vi "SERIAL_BufferLoopEx.vi"(11 "navX DevRef":T1={"SerialPortRef"={"DevStatus"={"status"=FALSE, "code"=0, "source"=""}, "Serial Port Name"=""}, "Board Information"={"WhoAmI (50 | 0x32)"=0, "Board Revision"=0, "Firmware Major Version"=0, "Firmware Minor Version"=0, "NAVX_BOARD_CAPABILITY"={"OMNIMOUNT"=FALSE, "YAW_RESET"=FALSE, "VEL_AND_DISP"=FALSE}, "NAVX_BOARD_YAW_AXIS"={"BOARD_YAW_AXIS_UP"=FALSE, "BOARD_YAW_AXIS"=0}}, "Status"={"Update Rate Hz"=0, "Accelerometer Full-Scale Range"=0, "Gyro Full-Scale Range"=0, "NAVX_OP_STATUS"=0, "NAVX_CAL_STATUS"=0, "NAVX_SELFTEST_STATUS"=0, "NAVX_SENSOR_STATUS"={"MOVING"=FALSE, "YAW_STABLE"=FALSE, "MAG_DISTURBANCE"=FALSE, "ALTITUDE_VALID"=FALSE, "SEALEVEL_PRESS_SET"=FALSE, "FUSED_HEADING_VALID"=FALSE}}, "Offsets"={"Yaw"=0.0, "Quat W"=0.0, "Quat X"=0.0, "Quat Y"=0.0, "Quat Z"=0.0}, "Update Rate (4Hz-60Hz)"=50, "Nav6Mode (YPR)"=enum."YPR", "refnum name"="", "error"={"status"=FALSE, "code"=0, "source"=""}, "Loop VI Refnum"=refnum, "Serial Port"=enum."Onboard RS-232"} {"Status"."NAVX_OP_STATUS" items=["INITIALIZING", "SELFTEST_IN_PROGRESS", "ERROR", "IMU_AUTOCAL_IN_PROGRESS", "NORMAL"]; "Status"."NAVX_CAL_STATUS" items=["IMU_CAL_STATE_MASK"=3, "IMU_CAL_INPROGRESS"=0, "IMU_CAL_ACCUMULATE"=1, "IMU_CAL_COMPLETE"=2, "MAG_CAL_COMPLETE"=4, "BARO_CAL_COMPLETE"=8]}) -> ()   [LabVIEW 2014, in "navX-MXP IMU.lvlib"]
uses:
  navX-MXP IMU.lvlib
  Internal/navX Serial DevRef.ctl
  <vilib>/Rock Robotics/WPI/SerialPort/WPI_SerialPortRef.ctl
  COMMON/TypeDefs/Data TypeDefs/navX Board Information.ctl
  COMMON/TypeDefs/Value TypeDefs/navX NAVX_BOARD_CAPABILITY.ctl
  COMMON/TypeDefs/Value TypeDefs/navX NAVX_BOARD_YAW_AXIS.ctl
  COMMON/TypeDefs/Data TypeDefs/navX Status Data.ctl
  COMMON/TypeDefs/Value TypeDefs/navX NAVX_OP_STATUS.ctl
  COMMON/TypeDefs/Value TypeDefs/navX NAVX_CAL_STATUS.ctl
  COMMON/TypeDefs/Value TypeDefs/navX NAVX_SENSOR_STATUS.ctl
  TypeDefs/navX Serial Mode.ctl
  NI WPI/WPI_SerialPort_USB.ctl
  TypeDefs/navX Data Packet ID.ctl
  <vilib>/Platform/TimedLoop/XDataNode/timing_clust.ctl
  <vilib>/Platform/TimedLoop/XDataNode/nitl_modes.ctl
  <vilib>/Platform/TimedLoop/XDataNode/wakeup.ctl
  TypeDefs/navxASCIIPacketHeaderTypes.ctl
  <vilib>/Rock Robotics/SystemInterfaces/Utilities/FPGA_UtilitiesRead LocalTime.vi
  <vilib>/platform/TimedLoop/XDataNode/XDataNode.xnode
  <vilib>/Platform/TimedLoop/XDataNode/XDNodeRunTimeDep.lvlib
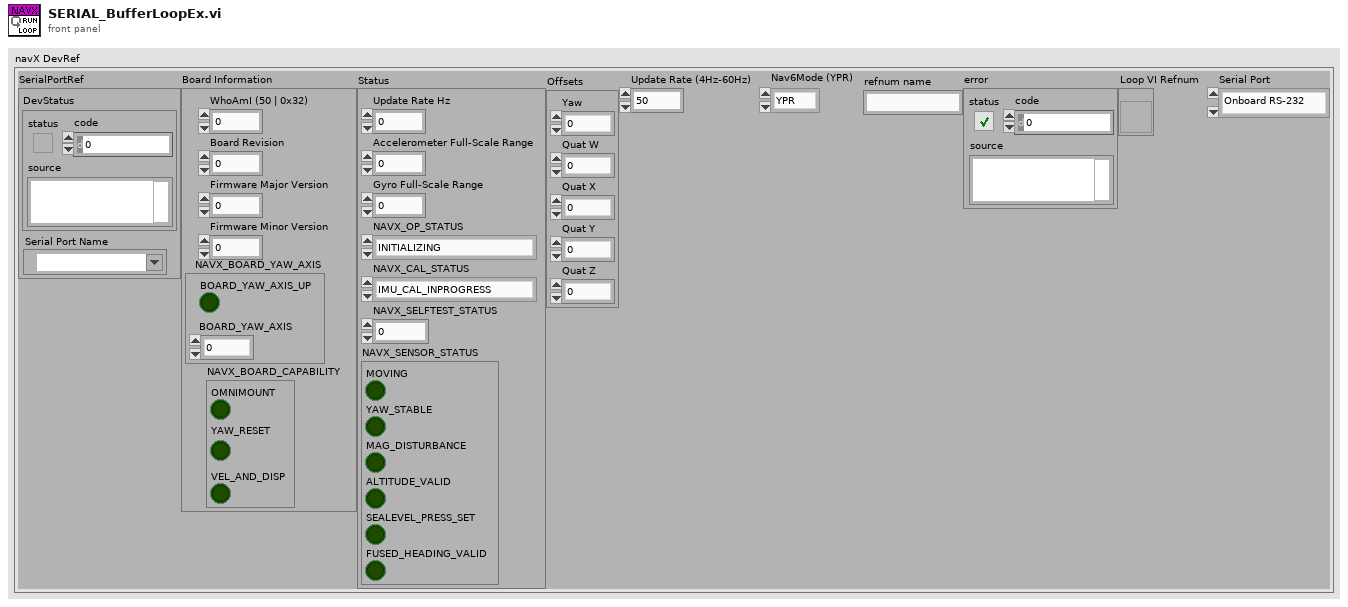
[diagram p1: front panel]
types:
  T1 = typedef "navX-MXP IMU.lvlib/navX Serial DevRef.ctl" = cluster{"SerialPortRef":T2, "Board Information":T3, "Status":T6, "Offsets":cluster{"Yaw":dbl, "Quat W":dbl, "Quat X":dbl, "Quat Y":dbl, "Quat Z":dbl}, "Update Rate (4Hz-60Hz)":u8, "Nav6Mode (YPR)":T10, "refnum name":string, "error":errorcluster, "Loop VI Refnum":refnum<vi>, "Serial Port":T11}
  T2 = typedef "WPI_SerialPortRef.ctl" = cluster{"DevStatus":errorcluster, "Serial Port Name":refnum<visa-resource-name>}
  T3 = typedef "navX-MXP IMU.lvlib/navX Board Information.ctl" = cluster{"WhoAmI (50 | 0x32)":u8, "Board Revision":u8, "Firmware Major Version":u8, "Firmware Minor Version":u8, "NAVX_BOARD_CAPABILITY":T4, "NAVX_BOARD_YAW_AXIS":T5}
  T4 = typedef "navX-MXP IMU.lvlib/navX NAVX_BOARD_CAPABILITY.ctl" = cluster{"OMNIMOUNT":bool, "YAW_RESET":bool, "VEL_AND_DISP":bool}
  T5 = typedef "navX-MXP IMU.lvlib/navX NAVX_BOARD_YAW_AXIS.ctl" = cluster{"BOARD_YAW_AXIS_UP":bool, "BOARD_YAW_AXIS":u8}
  T6 = typedef "navX-MXP IMU.lvlib/navX Status Data.ctl" = cluster{"Update Rate Hz":u8, "Accelerometer Full-Scale Range":u8, "Gyro Full-Scale Range":u16, "NAVX_OP_STATUS":T7, "NAVX_CAL_STATUS":T8, "NAVX_SELFTEST_STATUS":u8, "NAVX_SENSOR_STATUS":T9}
  T7 = typedef "navX-MXP IMU.lvlib/navX NAVX_OP_STATUS.ctl" = u8
  T8 = typedef "navX-MXP IMU.lvlib/navX NAVX_CAL_STATUS.ctl" = u8
  T9 = typedef "navX-MXP IMU.lvlib/navX NAVX_SENSOR_STATUS.ctl" = cluster{"MOVING":bool, "YAW_STABLE":bool, "MAG_DISTURBANCE":bool, "ALTITUDE_VALID":bool, "SEALEVEL_PRESS_SET":bool, "FUSED_HEADING_VALID":bool}
  T10 = typedef "navX-MXP IMU.lvlib/navX Serial Mode.ctl" = enum16{"YPR", "Gyro", "Quaternion", "AHRS", "AHRSPos"}
  T11 = typedef "navX-MXP IMU.lvlib/WPI_SerialPort_USB.ctl" = enum16{"Onboard RS-232", "MXP TTL", "USB"}
  T12 = typedef "navX Data Packet ID.ctl" = string[]
  T13 = typedef "XDNodeRunTimeDep.lvlib/timing_clust.ctl" = cluster{"Expected End [f-1]":u64, "Actual End [f-1]":u64, "Finished Late? [f-1]":bool, "Expected End [i-1]":u64, "Actual End [i-1]":u64, "Finished Late? [i-1]":bool, "Expected Start [i]":u64, "Actual Start [i]":u64, "Expected Start [f]":u64, "Actual Start [f]":u64, "Source Name":string, "Structure Name":string, "Period":i64, "Deadline":i64, "Offset":i64, "Start":i64, "Priority":i32, "Timeout":i32, "Mode":T14, "Wakeup Reason":T15, "Error":errorcluster, "Source Type":string, "Secondary Source Type":string, "Global End Time":u64, "Global Start Time":u64, "Frame Duration":u64, "Iteration Duration":u64, "Assigned CPU":i32, "I/O Scan Engine Mode":u32}
  T14 = typedef "XDNodeRunTimeDep.lvlib/nitl_modes.ctl" = enum32{"No Change", "Process missed periods, maintain original phase", "Discard missed periods, maintain original phase", "Process missed periods, ignore original phase", "Discard missed periods, ignore original phase"}
  T15 = typedef "XDNodeRunTimeDep.lvlib/wakeup.ctl" = enum32{"Normal", "Aborted", "Asynchronous wakeup", "Timing source error", "Timed loop error", "Timeout"}
  T16 = typedef "navX-MXP IMU.lvlib/navxASCIIPacketHeaderTypes.ctl" = string[]
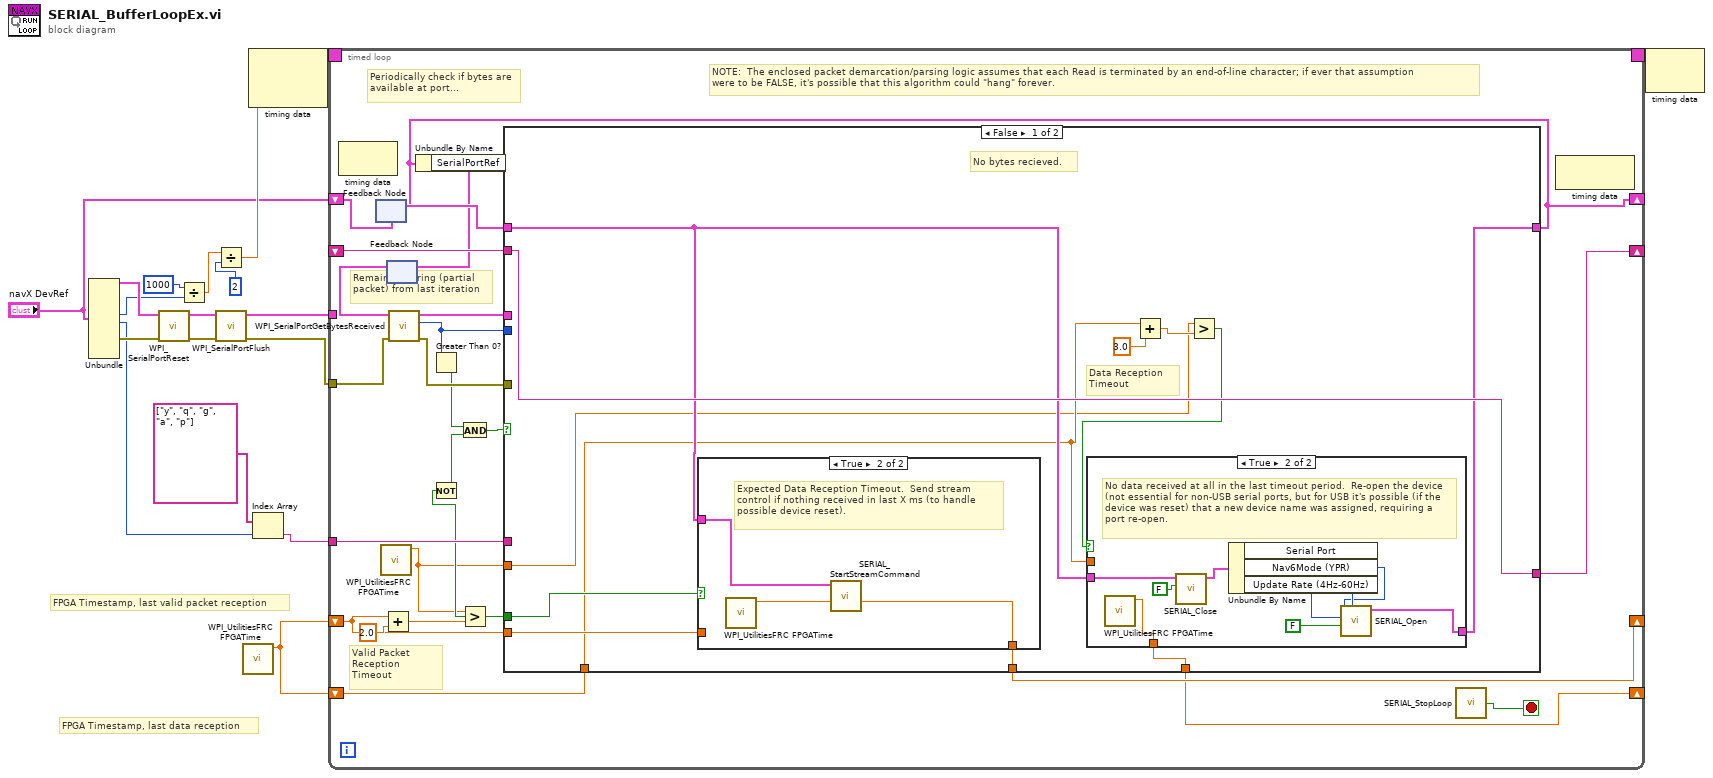
[diagram p0: block diagram]
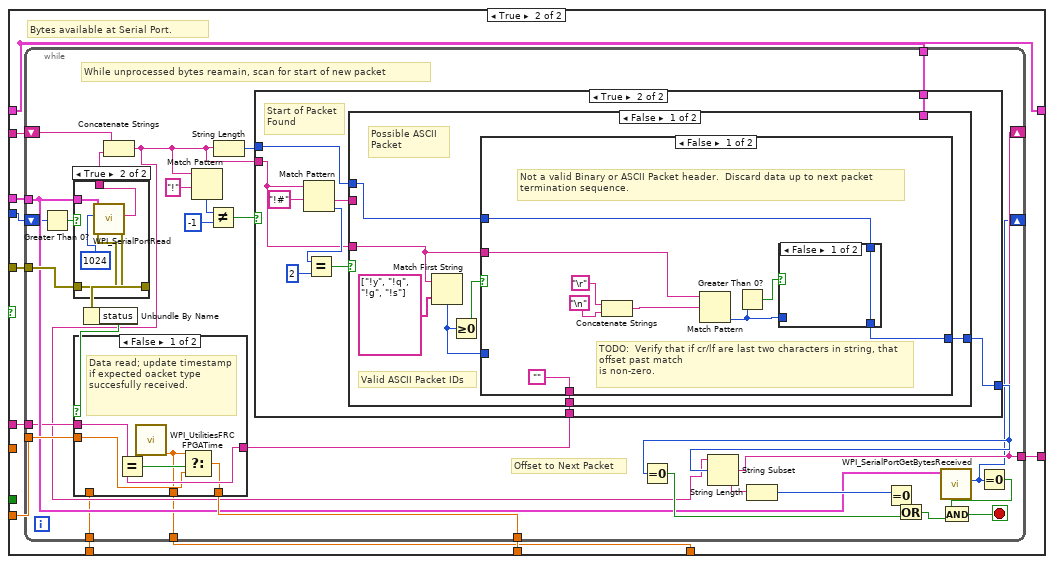
[diagram p4: hidden frame]
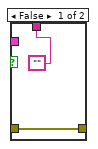
[diagram p5: hidden frame]
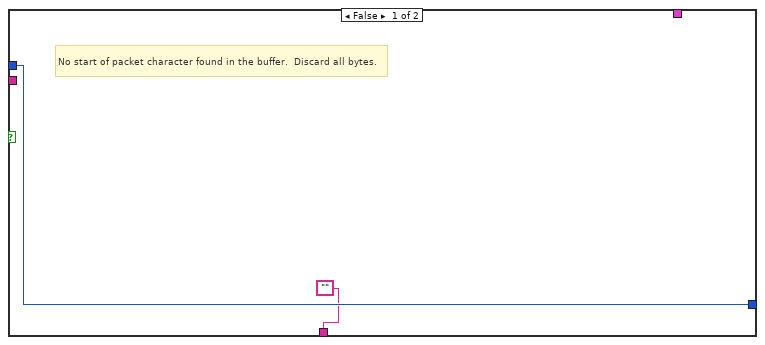
[diagram p7: hidden frame]
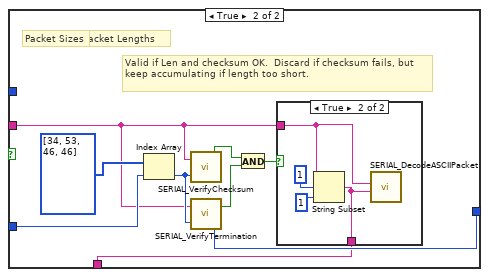
[diagram p9: hidden frame]
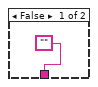
[diagram p10: hidden frame]
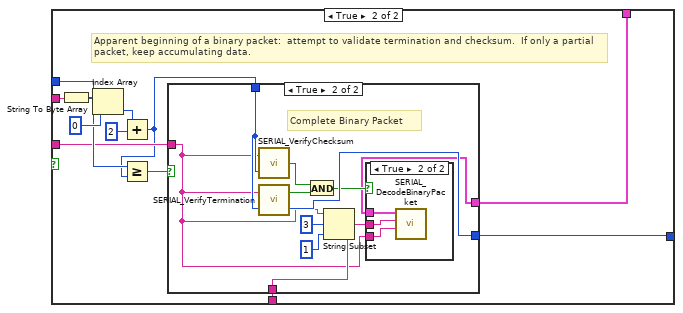
[diagram p11: hidden frame]
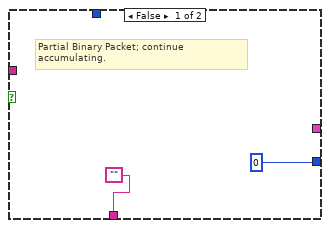
[diagram p12: hidden frame]
diagram:
  # "FPGA Timestamp, last data reception"
  # "FPGA Timestamp, last valid packet reception"
  n1 = Unbundle("navX DevRef") -> ("SerialPortRef"=w18:T2, "Update Rate (4Hz-60Hz)"=w12:u8, "Nav6Mode (YPR)"=w6:T10, "error"=w13:errorcluster)  [unwired: 6 out]
  n2 = call <vilib>:"WPI_SerialPortReset.vi"("error in (no error)"=w13, "SerialPortRef"=w18) -> ("error out"=w2:errorcluster, "SerialPortRef"=w1:T2)  [unwired: 8 in]
  n3 = Divide(x=1000, y=w12) -> (x/y=w10:dbl)
  n4 = Divide(x=w10, y=2) -> (x/y=w8:dbl)
  n5 = call <vilib>:"WPI_SerialPortFlush.vi"("error in (no error)"=w2, "SerialPortRef"=w1) -> ("error out"=w11:errorcluster, "SerialPortRef"=w14:T2)  [unwired: 8 in]
  n6 = call <vilib>:"WPI_UtilitiesFRC FPGATime.vi"() -> ("FPGA Time"=w4:dbl)  [unwired: 10 in, 1 out]
  n7 = node-c288(w8) -> (w17:T13)  [unwired: 1 in]
  n8 = Index Array(array=T12 ["y", "q", "g", "a", "p"], index=w6) -> (element=w5:string)
  n9 = timed-loop {
    timing: w17 -> [_]
    timing-out: [_] -> w16
    tunnel: w14 -> [_]
    tunnel: w11 -> [w37]
    shift-right: [w35] -> _
    shift-left: _ -> [w38]
    shift-right: [w36] -> _
    shift-left: w4 -> [w32]
    tunnel: w5 -> [w34]
    shift-right: [w26] -> _
    shift-left: w4 -> [w24]
    shift-right: [w21] -> _
    shift-left: "navX DevRef" -> [w22]
    stop <- w40 stop-if-true
    # "Valid Packet Reception Timeout"
    # "NOTE:  The enclosed packet demarcation/parsing logic assumes that each Read is terminated by an end-of-line character; if ever that assumption\nwere to be FALSE, it's possible that this algorithm could \"hang\" forever."
    # "Remainder string (partial packet) from last iteration"
    # "Periodically check if bytes are available at port..."
    n10 = node-c288() -> ()  [unwired: 1 in, 1 out]
    n11 = feedback #1(w22) -> (w39:T1)
    n12 = call <vilib>:"WPI_UtilitiesFRC FPGATime.vi"() -> ("FPGA Time"=w23:dbl)  [unwired: 10 in, 1 out]
    n13 = Add(x=w32, y=2.0) -> (x+y=w25:dbl)
    n14 = feedback #2() -> (w19:T2)  [unwired: 1 in]
    n15 = call <vilib>:"WPI_SerialPortGetBytesReceived.vi"("error in (no error)"=w37, "SerialPortRef"=w19) -> ("error out"=w41:errorcluster, "Bytes at Port"=w27:u32, "SerialPortRef"=w42:T2)  [unwired: 7 in]
    n16 = Greater Than 0?(x=w27) -> (x > 0?=w29:bool)
    n17 = Greater?(x=w23, y=w25) -> (0:w31:bool)
    n18 = Not(x=w31) -> (.not. x?=w30:bool)
    n19 = And(x=w29, y=w30) -> (x .and. y?=w28:bool)
    n20 = case shown="False" w28 {
      tunnel: w42 -> [_ w79]
      tunnel: w41 -> [_ w78]
      tunnel: w39 -> [w49 w72]
      tunnel: [w48 w72] -> w21
      tunnel: [w51 w77] -> w35
      tunnel: w38 -> [w51 w75]
      tunnel: [w53 w71] -> w36
      tunnel: w32 -> [w52 w76]
      tunnel: w34 -> [_ w74]
      tunnel: w31 -> [w54 _]
      tunnel: w27 -> [_ w73]
      tunnel: [w50 w70] -> w26
      tunnel: w24 -> [w45 w69]
      tunnel: w23 -> [w43 _]
      frame False {
        # "Data Reception Timeout"
        # "No bytes recieved."
        n21 = case shown="True" w54 {
          tunnel: w49 -> [_ w68]
          tunnel: [w66 w67] -> w53
          tunnel: w52 -> [w66 _]
          frame False {
          }
          frame True {
            # "Expected Data Reception Timeout.  Send stream control if nothing received in last X ms (to handle possible device reset)."
            n22 = call <vilib>:"WPI_UtilitiesFRC FPGATime.vi"() -> ("FPGA Time"=w67:dbl)  [unwired: 10 in, 1 out]
            n23 = call "SERIAL_StartStreamCommand.vi"("navX Ref"=w68) -> ()  [unwired: 10 in, 1 out]
          }
        }
        n24 = Add(x=w45, y=3.0) -> (x+y=w47:dbl)
        n25 = Greater?(x=w43, y=w47) -> (0:w44:bool)
        n26 = case shown="True" w44 {
          tunnel: w49 -> [w55 w64]
          tunnel: w45 -> [w56 _]
          tunnel: [w56 w65] -> w50
          tunnel: [w55 w57] -> w48
          frame False {
          }
          frame True {
            # "No data received at all in the last timeout period.  Re-open the device (not essential for non-USB serial ports, but for USB it's possible (if the device was reset) that a new device name was assigned, requiring a port re-open."
            n27 = call <vilib>:"WPI_UtilitiesFRC FPGATime.vi"() -> ("FPGA Time"=w65:dbl)  [unwired: 10 in, 1 out]
            n28 = call "SERIAL_Close.vi"("StopLoop"=FALSE, "navX DevRef"=w64) -> ("navX DevRef"=w62:T1)  [unwired: 8 in, 1 out]
            n29 = Unbundle By Name(w62) -> ("Serial Port"=w61:T11, "Nav6Mode (YPR)"=w60:T10, "Update Rate (4Hz-60Hz)"=w59:u8)
            n30 = call "SERIAL_Open.vi"("Serial Port (MXP)"=w61, "CreateNewLoop"=FALSE, "Update Rate (4Hz-60Hz)"=w59, "Nav6Mode (YPR)"=w60) -> ("navX Ref"=w57:T1)  [unwired: 5 in, 2 out]
          }
        }
      }
      frame True {
        # "Bytes available at Serial Port."
        n31 = while {
          tunnel: w79 -> [w93]
          tunnel: w78 -> [w99]
          tunnel: [w88] -> w77
          tunnel: [w96] -> w71
          tunnel: w76 -> [w95]
          tunnel: w72 -> [w94]
          shift-right: [w88] -> _
          shift-left: w75 -> [w89]
          tunnel: w74 -> [w87]
          shift-right: [w85] -> _
          shift-left: w73 -> [w84]
          tunnel: [w81] -> w70
          tunnel: w69 -> [w80]
          stop <- w90 stop-if-true
          # "Offset to Next Packet"
          # "While unprocessed bytes reamain, scan for start of new packet"
          n32 = Greater Than 0?(x=w84) -> (x > 0?=w83:bool)
          n33 = case shown="True" w83 {
            tunnel: ["" w116] -> w104
            tunnel: w99 -> [w110 w114]
            tunnel: [w110 w113] -> w98
            tunnel: w93 -> [_ w112]
            frame False {
            }
            frame True {
              n34 = call <vilib>:"WPI_SerialPortRead.vi"("error in (no error)"=w114, "Num Bytes to Read"=1024, "SerialPortRef"=w112) -> ("error out"=w113:errorcluster, "Buffer"=w116:string)  [unwired: 6 in, 1 out]
            }
          }
          n35 = Unbundle By Name(w98) -> ("status"=w97:bool)
          n36 = Concatenate Strings(w89, w104) -> (w82:string)
          n37 = Match Pattern(string=w82, regular expression="!") -> (offset past match=w108:i32)  [unwired: 1 in, 3 out]
          n38 = Not Equal?(x=w108, y=-1) -> (x != y?=w105:bool)
          n39 = String Length(string=w82) -> (length=w106:i32)
          n40 = case shown="True" w105 {
            tunnel: w106 -> [w126 w133]
            tunnel: w82 -> [_ w131]
            tunnel: [w126 w130] -> w103
            tunnel: w94 -> [_ w129]
            tunnel: ["" w127] -> w86
            frame False {
              # "No start of packet character found in the buffer.  Discard all bytes."
            }
            frame True {
              # "Start of Packet\nFound"
              n41 = Match Pattern(string=w131, regular expression="!#") -> (after substring=w128:string, offset past match=w135:i32)  [unwired: 1 in, 2 out]
              n42 = Equal?(x=w135, y=2) -> (x = y?=w132:bool)
              n43 = case shown="False" w132 {
                tunnel: w128 -> [_ w180]
                tunnel: w133 -> [w140 w177]
                tunnel: w131 -> [w142 w173]
                tunnel: [w138 w172] -> w130
                tunnel: w129 -> [_ w171]
                tunnel: [w137 w170] -> w127
                frame False {
                  # "Possible ASCII \nPacket"
                  # "Valid ASCII Packet IDs"
                  n44 = Match First String(2:T16 ["!y", "!q", "!g", "!s"], 3:w142) -> (0:w141:i32)  [unwired: 1 out]
                  n45 = Greater Or Equal To 0?(x=w141) -> (x >= 0?=w139:bool)
                  n46 = case shown="False" w139 {
                    tunnel: w142 -> [w150 w158]
                    tunnel: w141 -> [_ w163]
                    tunnel: w140 -> [w145 _]
                    tunnel: [w146 w159] -> w138
                    tunnel: ["" w156] -> w137
                    frame False {
                      # "TODO:  Verify that if cr/lf are last two characters in string, that offset past match\nis non-zero."
                      # "Not a valid Binary or ASCII Packet header.  Discard data up to next packet\ntermination sequence."
                      n47 = Concatenate Strings("\r", "\n") -> (w149:string)
                      n48 = Match Pattern(string=w150, regular expression=w149) -> (offset past match=w147:i32)  [unwired: 1 in, 3 out]
                      n49 = Greater Than 0?(x=w147) -> (x > 0?=w148:bool)
                      n50 = case shown="False" w148 {
                        tunnel: w147 -> [_ w154]
                        tunnel: [w153 w154] -> w146
                        tunnel: w145 -> [w153 _]
                        frame False {
                        }
                        frame True {
                        }
                      }
                    }
                    frame True {
                      # "Valid if Len and checksum OK.  Discard if checksum fails, but keep accumulating if length too short."
                      # "Valid ASCII Packet Lengths"
                      # "Packet Sizes"
                      n51 = Index Array(array=i32[] [34, 53, 46, 46], index=w163) -> (element=w161:i32)
                      n52 = call "SERIAL_VerifyChecksum.vi"("ExpectedFullPacketLength"=w161, "Packet\n\n\n\n\n\n\n\n\n\n\n\n\n\nPacketContent"=w158) -> ("Valid Checksum"=w155:bool)
                      n53 = call "SERIAL_VerifyTermination.vi"("ExpectedFullPacketLength"=w161, "Packet\n\n\n\n\n\n\n\n\n\n\n\n\n\nPacketContent"=w158) -> ("OffsetPastTermination"=w159:i32, "ValidTermination"=w160:bool)
                      n54 = And(x=w155, y=w160) -> (x .and. y?=w157:bool)
                      n55 = case shown="True" w157 {
                        tunnel: w158 -> [_ w166]
                        tunnel: ["" w165] -> w156
                        frame False {
                        }
                        frame True {
                          n56 = String Subset(string=w166, offset (0)=1, length (rest)=1) -> (substring=w165:string)
                          n57 = call "SERIAL_DecodeASCIIPacket.vi"("PacketType"=w165, "Buffer"=w166) -> ()  [unwired: 7 in, 3 out]
                        }
                      }
                    }
                  }
                }
                frame True {
                  # "Apparent beginning of a binary packet:  attempt to validate termination and checksum.  If only a partial packet, keep accumulating data."
                  n58 = String To Byte Array(string=w180) -> (unsigned byte array=w179:u8[])
                  n59 = Index Array(array=w179, index=0) -> (element=w175:u8)
                  n60 = Add(x=w175, y=2) -> (x+y=w169:i32)
                  n61 = Greater Or Equal?(x=w177, y=w169) -> (x >= y?=w176:bool)
                  n62 = case shown="True" w176 {
                    tunnel: w173 -> [_ w183]
                    tunnel: w169 -> [_ w192]
                    tunnel: [0 w189] -> w172
                    tunnel: w171 -> [_ w185]
                    tunnel: ["" w184] -> w170
                    frame False {
                      # "Partial Binary Packet; continue accumulating."
                    }
                    frame True {
                      # "Complete Binary Packet"
                      n63 = call "SERIAL_VerifyChecksum.vi"("ExpectedFullPacketLength"=w192, "Packet\n\n\n\n\n\n\n\n\n\n\n\n\n\nPacketContent"=w183) -> ("Valid Checksum"=w191:bool)
                      n64 = call "SERIAL_VerifyTermination.vi"("ExpectedFullPacketLength"=w192, "Packet\n\n\n\n\n\n\n\n\n\n\n\n\n\nPacketContent"=w183) -> ("OffsetPastTermination"=w189:i32, "ValidTermination"=w190:bool)
                      n65 = And(x=w191, y=w190) -> (x .and. y?=w186:bool)
                      n66 = String Subset(string=w183, offset (0)=3, length (rest)=1) -> (substring=w184:string)
                      n67 = case shown="True" w186 {
                        tunnel: w183 -> [_ w194]
                        tunnel: w184 -> [_ w195]
                        tunnel: w185 -> [_ w193]
                        frame False {
                          # "Corrupted\nPacket;\ndiscard"
                        }
                        frame True {
                          n68 = call "SERIAL_DecodeBinaryPacket.vi"("navX DevRef"=w193, "PacketType"=w195, "Buffer"=w194) -> ()  [unwired: 7 in, 1 out]
                        }
                      }
                    }
                  }
                }
              }
            }
          }
          n69 = case shown="False" w97 {
            tunnel: [w118 w124] -> w96
            tunnel: w95 -> [w119 w124]
            tunnel: w87 -> [w122 _]
            tunnel: w86 -> [w121 _]
            tunnel: [w117 w123] -> w81
            tunnel: w80 -> [_ w123]
            frame False {
              # "Data read; update timestamp if expected oacket type  succesfully received."
              n70 = Equal?(x=w122, y=w121) -> (x = y?=w120:bool)
              n71 = call <vilib>:"WPI_UtilitiesFRC FPGATime.vi"() -> ("FPGA Time"=w117:dbl)  [unwired: 10 in, 1 out]
              n72 = Select(t=w117, s=w120, f=w119) -> (s? t:f=w118:dbl)
            }
            frame True {
              # "Error reading\ndata. at port."
            }
          }
          n73 = Equal To 0?(x=w103) -> (x = 0?=w100:bool)
          n74 = String Subset(string=w82, offset (0)=w103) -> (substring=w88:string)  [unwired: 1 in]
          n75 = String Length(string=w88) -> (length=w102:i32)
          n76 = Equal To 0?(x=w102) -> (x = 0?=w101:bool)
          n77 = Or(x=w101, y=w100) -> (x .or. y?=w92:bool)
          n78 = call <vilib>:"WPI_SerialPortGetBytesReceived.vi"("SerialPortRef"=w93) -> ("Bytes at Port"=w85:u32)  [unwired: 8 in, 2 out]
          n79 = Equal To 0?(x=w85) -> (x = 0?=w91:bool)
          n80 = And(x=w91, y=w92) -> (x .and. y?=w90:bool)
        }
      }
    }
    n81 = feedback-in #1(w21) -> ()
    n82 = Unbundle By Name(w21) -> ("SerialPortRef"=w20:T2)
    n83 = feedback-in #2(w20) -> ()
    n84 = call "SERIAL_StopLoop.vi"() -> ("Stop?"=w40:bool)  [unwired: 2 in]
    n85 = node-c288() -> ()  [unwired: 1 in, 1 out]
  }
  n86 = node-c288(w16) -> ()  [unwired: 1 out]
